vi "Test Failing Test.vi"(8 "error in (no error)":errorcluster, 11 "LUnit Test Case V2 Test Double in":refnum<class "Light Test Case Double.lvclass">) -> (0 "error out":errorcluster, 3 "LUnit Test Case V2 Test Double out":refnum<class "Light Test Case Double.lvclass">)   [LabVIEW 2020, in "Light Test Case Double.lvclass"]
uses:
  Light Test Case Double.lvclass
  C:/git/astemes-lunit/source/Core/LUnit Test Case/LUnit Test Case.lvclass
  source/API/LUnit Test Case/LUnit Test Case.lvclass/LUnit Test Case.ctl
  source/API/LUnit Test Case/Private/Append Fail Result.vi
  Light Test Case Double.lvclass/Light Test Case Double.ctl
  source/API/LUnit Test Case/LUnit Test Case.lvclass
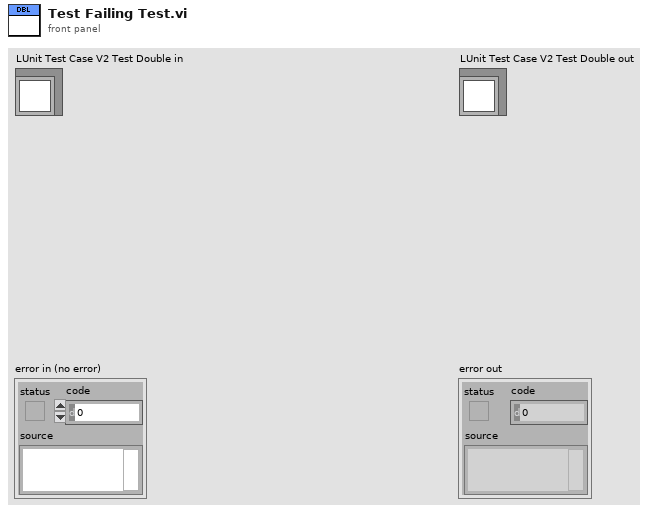
[diagram p1: front panel]
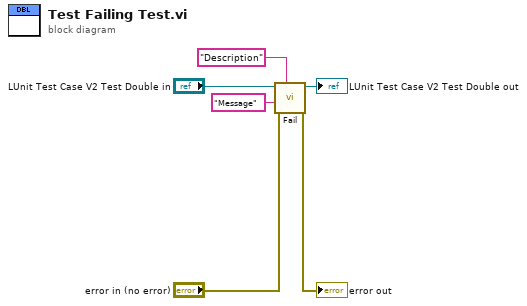
[diagram p0: block diagram]
diagram:
  n1 = call "Fail.vi"("Description"="Description", "error in (no error)"="error in (no error)", "Message"="Message", "LUnit Test Case In"="LUnit Test Case V2 Test Double in") -> ("error out"=→"error out":errorcluster, "LUnit Test Case Out"=→"LUnit Test Case V2 Test Double out":refnum<class "Light Test Case Double.lvclass">)  [unwired: 6 in]
